vi "Init Digitizers.vi"(6 "NI Cards":i32=3, 8 "Bypass 2nd Digitizer Init":bool, 9 "Digitizer Config":T3=enum."5-CH pulser w/ ann array", 10 "Main Digitizer":T2=enum."NI Digitizer", 11 "Digitizer Settings in":T1={"Digitizer delay (us) "=0.0, "rf points per line"=0, "lines per plane"=0, "Samp Rate (Hz)"=0.0, "Additional dig delay (us)"=0.0, "Voltage Scale"=0.0, "Pre-Looks"=0, "Offset delay (us)"=0.0, "bits A/D"=0, "Avg Num"=0, "DigTimeOut"=0.0, "Rel Dig Delay"=0.0, "Dig Ch"=0, "LeCroyCluster"={"LeCroy Channels"=[], "LC read pt offset"=0.0, "Sweep Avg"=FALSE}, "Main Digitizer"=enum."Acqiris Digitizer", "Dig Config"=enum."Single channel", "Digitizer ID Cluster"={"Acqiris/Alazar/SP ID"=[], "NI Instr Handles"=[], "LeCroy VISA"="", "GaGe Handle"={"Handle"=0, "Sample size"=0, "Resolution"=0, "Offset"=0, "Channels"=0, "Boards"=0}, "ATS Ref"="", "Acqiris Address"=[], "ADQRef"=refnum, "adq_cu_ptr"=refnum}, "Trigger Settings"={"Trig Source"=0, "Trig Coupling"=0, "Trig Slope"=0, "Level (mV)"=0.0}, "Bulk Acq"=FALSE, "Bulk Start Indexes"=[], "Data Ref RF"=refnum, "NI ID/Channel"=[], "Total Dig CH"=1, "Xtra Ann Trig delay (us)"=10.0, "Fix Z Delay?"=FALSE, "One Way Transmission?"=FALSE, "Data Ref Log"=refnum} {"Trigger Settings"."Trig Slope" items=["Positive", "Negative"]; "Trigger Settings"."Level (mV)" format="%.2f"; "Trigger Settings"."Trig Coupling" items=["DC 1 MOhm", "AC 1 MOhm", "DC 50 Ohm", "AC 50 Ohm"]; "Trigger Settings"."Trig Source" items=["Chan 1", "External"]; "Rel Dig Delay" format="%.2f"; "DigTimeOut" format="%.2f"; "Avg Num" min=1; "Offset delay (us)" format="%.2f"; "Additional dig delay (us)" format="%.2f"; "Digitizer delay (us)" format="%.2f"}) -> (0 "Bypass 2nd Digitizer Init":bool, 1 "Initialization Failed!!":bool, 3 "Digitizer Settings":T1={"Digitizer delay (us) "=0.0, "rf points per line"=0, "lines per plane"=0, "Samp Rate (Hz)"=0.0, "Additional dig delay (us)"=0.0, "Voltage Scale"=0.0, "Pre-Looks"=0, "Offset delay (us)"=0.0, "bits A/D"=0, "Avg Num"=0, "DigTimeOut"=0.0, "Rel Dig Delay"=0.0, "Dig Ch"=0, "LeCroyCluster"={"LeCroy Channels"=[], "LC read pt offset"=0.0, "Sweep Avg"=FALSE}, "Main Digitizer"=enum."Acqiris Digitizer", "Dig Config"=enum."Single channel", "Digitizer ID Cluster"={"Acqiris/Alazar/SP ID"=[], "NI Instr Handles"=[], "LeCroy VISA"="", "GaGe Handle"={"Handle"=0, "Sample size"=0, "Resolution"=0, "Offset"=0, "Channels"=0, "Boards"=0}, "ATS Ref"="", "Acqiris Address"=[], "ADQRef"=refnum, "adq_cu_ptr"=refnum}, "Trigger Settings"={"Trig Source"=0, "Trig Coupling"=0, "Trig Slope"=0, "Level (mV)"=0.0}, "Bulk Acq"=FALSE, "Bulk Start Indexes"=[], "Data Ref RF"=refnum, "NI ID/Channel"=[], "Total Dig CH"=1, "Xtra Ann Trig delay (us)"=10.0, "Fix Z Delay?"=FALSE, "One Way Transmission?"=FALSE, "Data Ref Log"=refnum} {"Trigger Settings"."Trig Slope" items=["Positive", "Negative"]; "Trigger Settings"."Level (mV)" format="%.2f"; "Trigger Settings"."Trig Coupling" items=["DC 1 MOhm", "AC 1 MOhm", "DC 50 Ohm", "AC 50 Ohm"]; "Trigger Settings"."Trig Source" items=["Chan 1", "External"]; "Rel Dig Delay" format="%.2f"; "DigTimeOut" format="%.2f"; "Avg Num" min=1; "Offset delay (us)" format="%.2f"; "Additional dig delay (us)" format="%.2f"; "Digitizer delay (us)" format="%.2f"})   [LabVIEW 2022 SP3]
uses:
  -DigitizerRoutines/Digitizer.ctl
  -DigitizerRoutines/DigConfig.ctl
  -DigitizerRoutines/DigitizerSettings.ctl
  -DigitizerRoutines/DigitizerID.ctl
  C:/Windows/System32/ADQAPI_dotNet_helper.dll
  <instrlib>/niScope/Controls/niScope input clock source.ctl
  <instrlib>/Acqiris Dx/Acqiris Dx.lvlib
  <instrlib>/Acqiris Bx/Acqiris Bx.lvlib
  <instrlib>/LeCroy Wave Series/LeCroy Wave Series.lvlib
panel:
  out "error out":errorcluster
  in  "error in (no error)":errorcluster
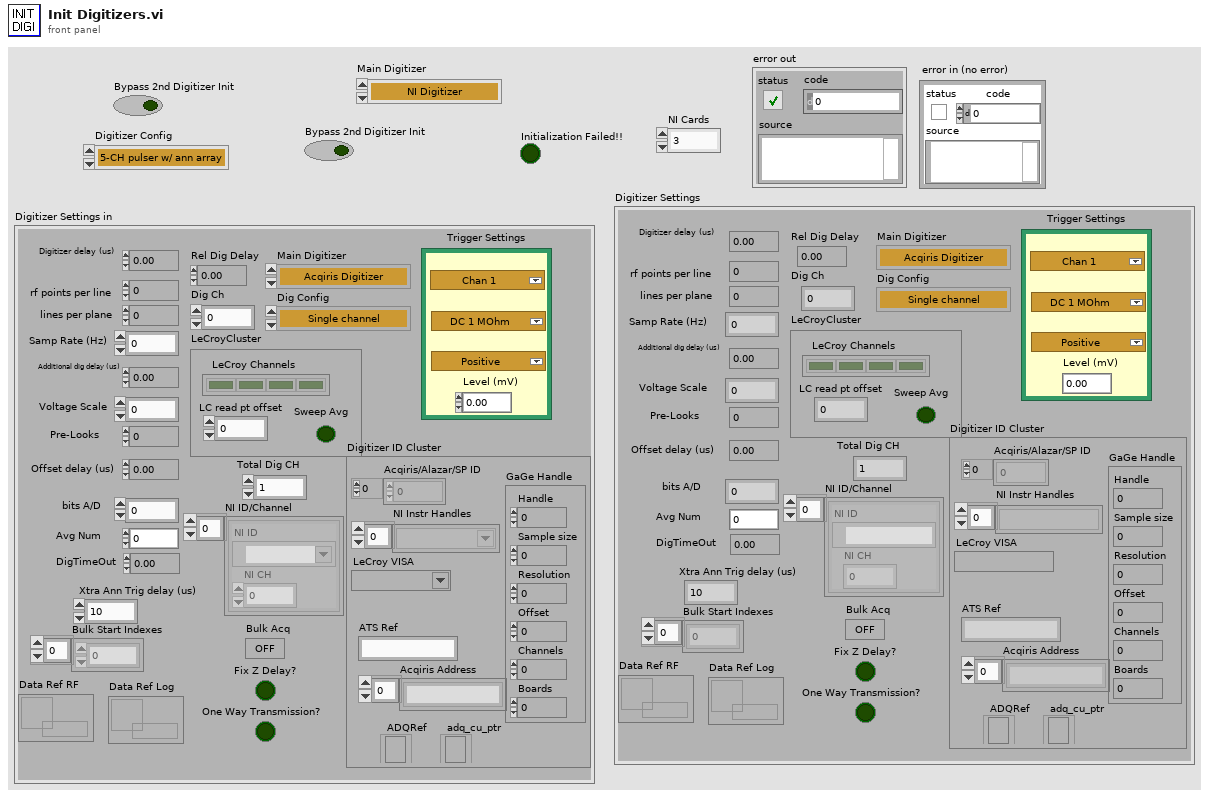
[diagram p1: front panel]
types:
  T1 = typedef "DigitizerSettings.ctl" = cluster{"Digitizer delay (us) ":dbl, "rf points per line":i32, "lines per plane":i32, "Samp Rate (Hz)":dbl, "Additional dig delay (us)":dbl, "Voltage Scale":dbl, "Pre-Looks":i32, "Offset delay (us)":dbl, "bits A/D":i8, "Avg Num":i32, "DigTimeOut":sgl, "Rel Dig Delay":sgl, "Dig Ch":i32, "LeCroyCluster":cluster{"LeCroy Channels":bool[], "LC read pt offset":dbl, "Sweep Avg":bool}, "Main Digitizer":T2, "Dig Config":T3, "Digitizer ID Cluster":T4, "Trigger Settings":cluster{"Trig Source":u16, "Trig Coupling":u16, "Trig Slope":u16, "Level (mV)":dbl}, "Bulk Acq":bool, "Bulk Start Indexes":i32[], "Data Ref RF":refnum<data-value>, "NI ID/Channel":cluster{"NI ID":refnum<k15>, "NI CH":i32}[], "Total Dig CH":i32, "Xtra Ann Trig delay (us)":dbl, "Fix Z Delay?":bool, "One Way Transmission?":bool, "Data Ref Log":refnum<data-value>}
  T2 = typedef "Digitizer.ctl" = enum16{"Acqiris Digitizer", "NI Digitizer", "LeCroy", "GaGe", "AlazarTech", "No Digitizer", "Teledyne"}
  T3 = typedef "DigConfig.ctl" = enum16{"Single channel", "2 Chans w/ 2 Acqiris", "2 Chans w/ 1 Acqiris", "5-CH Pulser New", "5-CH pulser w/ ann array", "5-pass style ann array", "Empty"}
  T4 = typedef "DigitizerID.ctl" = cluster{"Acqiris/Alazar/SP ID":u32[], "NI Instr Handles":refnum<k15>[], "LeCroy VISA":refnum<visa-resource-name>, "GaGe Handle":cluster{"Handle":u32, "Sample size":u32, "Resolution":i32, "Offset":i32, "Channels":u32, "Boards":u32}, "ATS Ref":string, "Acqiris Address":string[], "ADQRef":refnum<k24>, "adq_cu_ptr":refnum<k24>}
  T5 = typedef "niScope input clock source.ctl" = u16
  T6 = cluster{"instrument handle out":refnum<k15>, i32}
  T7 = cluster{"instrument handle out":refnum<k15>, i32}[]
  T8 = cluster{"Handle":u32, "Sample size":u32, "Resolution":i32, "Offset":i32, "Channels":u32, "Boards":u32}
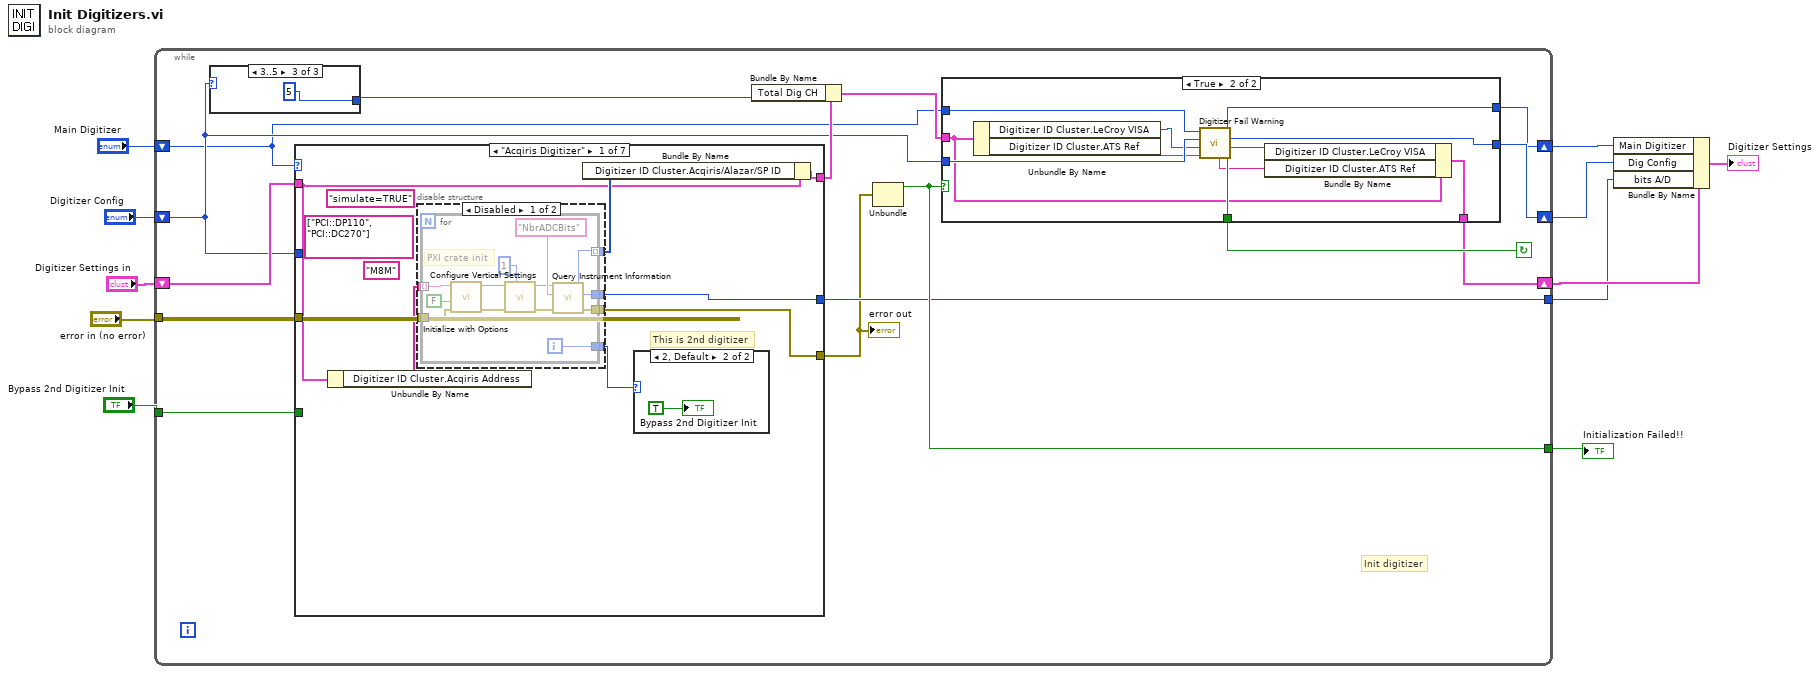
[diagram p0: block diagram]
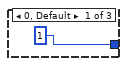
[diagram p2: hidden frame]
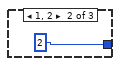
[diagram p3: hidden frame]
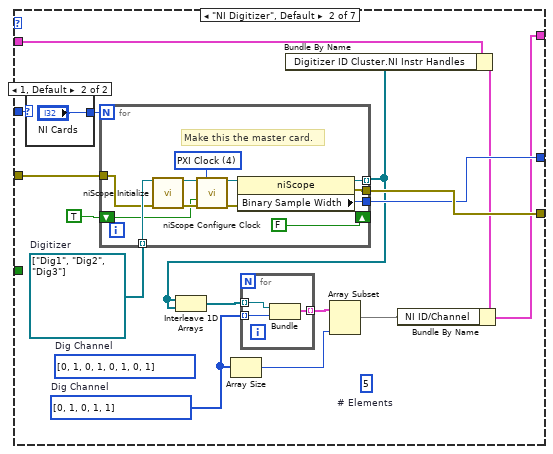
[diagram p7: hidden frame]
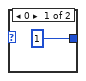
[diagram p8: hidden frame]
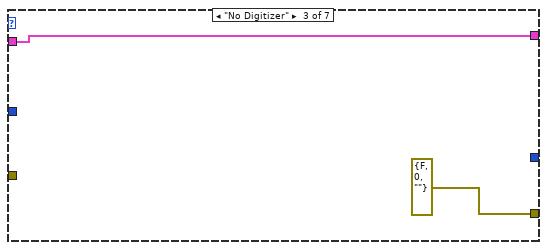
[diagram p9: hidden frame]
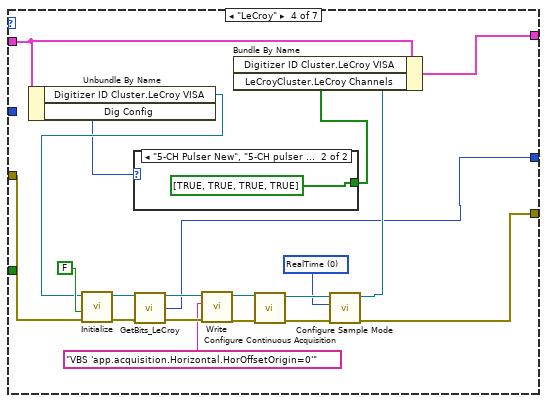
[diagram p10: hidden frame]
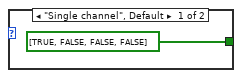
[diagram p11: hidden frame]
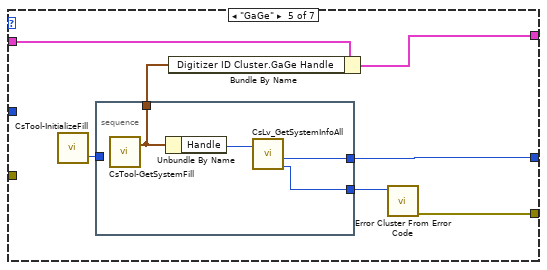
[diagram p12: hidden frame]
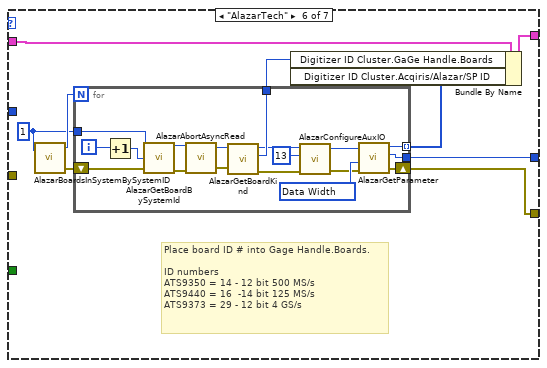
[diagram p13: hidden frame]
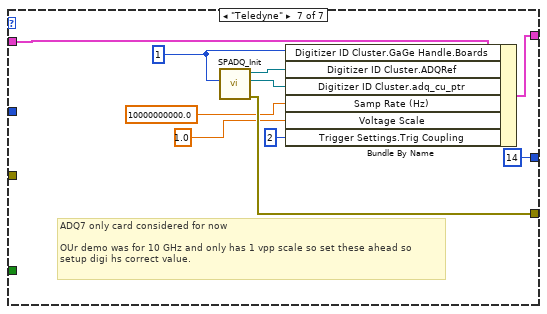
[diagram p14: hidden frame]
diagram:
  n1 = while {
    tunnel: "Bypass 2nd Digitizer Init" -> [w26]
    tunnel: "error in (no error)" -> [w24]
    tunnel: [w23] -> w8
    shift-right: [w17] -> w5
    shift-left: "Digitizer Settings in" -> [w25]
    shift-right: [w21] -> w2
    shift-left: "Digitizer Config" -> [w13]
    shift-right: [w20] -> w3
    shift-left: "Main Digitizer" -> [w12]
    tunnel: [w19] -> w1
    stop <- w22 continue-if-true
    # "Init digitizer"
    n2 = case shown="3..5" w13 {
      tunnel: [1 2 5] -> w14
      frame 0, Default {
      }
      frame 1, 2 {
      }
      frame 3..5 {
      }
    }
    n3 = case shown="\"Acqiris Digitizer\"" w12 {
      tunnel: [w50 w83 _ w110 w136 w146 u32 14 ("Sample Bits")] -> w19
      tunnel: w26 -> [_ _ _ _ _ _ _]
      tunnel: w13 -> [_ w88 _ _ _ _ _]
      tunnel: w25 -> [w49 w86 w106 w114 w134 w148 w175]
      tunnel: [w52 w78 w106 w115 w130 w149 w177] -> w16
      tunnel: [w47 w85 errorcluster {"status"=FALSE, "code"=0, "source"=""} ("error IO") w112 w131 w147 w171] -> w18
      tunnel: w24 -> [w46 w84 _ w113 _ _ _]
      frame "Acqiris Digitizer" {
        (unwired) "M8M" ("Options String (null string)")
        (unwired) string[] ["PCI::DP110", "PCI::DC270"]
        (unwired) "simulate=TRUE" ("Options String (null string)")
        # "This is 2nd digitizer"
        n4 = Unbundle By Name(w49) -> ("Digitizer ID Cluster.Acqiris Address"=w48:string[])
        n5 = disable-structure shown="Disabled" {
          disable-tunnel: [w58 _] -> w51
          disable-tunnel: [w57 _] -> w50
          disable-tunnel: w48 -> [w56 _]
          disable-tunnel: [w55 _] -> w47
          disable-tunnel: w46 -> [w54 _]
          disable-tunnel: [w53 _] -> w45
          frame Disabled {
            n6 = for {
              tunnel: [w64] -> w58 mode=indexing
              tunnel: w56 -> [w67] mode=indexing
              tunnel: [w62] -> w57
              tunnel: [w61] -> w55
              tunnel: w54 -> [w60]
              tunnel: [w59] -> w53
              i -> [w59]
              # "PXI crate init"
              n7 = call <instrlib>:"Initialize with Options.vi"("Resource Name (PCI::INSTR0)"=w67, "Reset (T: Reset)"=FALSE, "error in (no error)"=w60) -> ("Instrument ID"=w70:u32, "error out"=w69:errorcluster)  [unwired: 3 in, 2 out]
              n8 = call <instrlib>:"Configure Vertical Settings.vi"("Channel (1)"=1, "error in (no error)"=w69, "Instrument ID"=w70) -> ("error out"=w63:errorcluster, "dup Instrument ID"=w65:u32)  [unwired: 4 in, 3 out]
              n9 = call <instrlib>:"Query Instrument Information.vi"("Instrument ID"=w65, "Parameter String"="NbrADCBits", "error in (no error)"=w63) -> ("dup Instrument ID"=w64:u32, "Info Value (I32)"=w62:i32, "error out"=w61:errorcluster)  [unwired: 1 in, 3 out]
            }
          }
          frame Enabled {
          }
        }
        n10 = Bundle By Name(cluster=w49, "Digitizer ID Cluster.Acqiris/Alazar/SP ID"=w51) -> (w52:T1)
        n11 = case shown="2, Default" w45 {
          frame 0, 1 {
          }
          frame 2, Default {
            "Bypass 2nd Digitizer Init" <- TRUE ("Bypass 2nd Digitizer Init")
          }
        }
      }
      frame "NI Digitizer", Default {
        w73 = i32[] [0, 1, 0, 1, 1]  # Dig Channel
        (unwired) 5  # # Elements
        (unwired) i32[] [0, 1, 0, 1, 0, 1, 0, 1]  # Dig Channel
        w82 = refnum<k15>[] ["Dig1", "Dig2", "Dig3"]  # Digitizer
        n12 = case shown="1, Default" w88 {
          tunnel: [1 "NI Cards"] -> w87
          frame 0 {
          }
          frame 1, Default {
          }
        }
        n13 = for {
          N: w87 -> [_]
          tunnel: [w101] -> w74 mode=indexing
          tunnel: [w99] -> w83
          tunnel: w82 -> [w98] mode=indexing
          tunnel: [w97] -> w85
          tunnel: w84 -> [w96]
          shift-right: [FALSE] -> _
          shift-left: TRUE -> [w94]
          w103 = T5 4 items=["None"=0, "RTSI Clock"=1, "PFI 0"=6, "PFI 1"=2, "PFI 2"=3, "PXI Clock"=4, "External"=5, "Clock In"=7] ("input clock source")
          # "Make this the master card."
          n14 = call <instrlib>:"niScope Initialize.vi"("resource name"=w98, "error in"=w96) -> ("instrument handle"=w105:refnum<k15>, "error out"=w104:errorcluster)  [unwired: 2 in, 10 out]
          n15 = call <instrlib>:"niScope Configure Clock.vi"("instrument handle"=w105, "input clock source"=w103, "master enabled"=w94, "error in"=w104) -> ("instrument handle out"=w102:refnum<k15>, "error out"=w100:errorcluster)  [unwired: 2 in, 8 out]
          n16 = property class="niScope"(reference=w102, error in=w100) -> (reference out=w101:refnum<k15>, error out=w97:errorcluster, "Binary Sample Width"=w99:i32)
        }
        n17 = Interleave 1D Arrays(w74, w74) -> (w75:refnum<k15>[])
        n18 = Array Size(array=w73) -> (size(s)=w76:i32)
        n19 = for {
          tunnel: w75 -> [w91] mode=indexing
          tunnel: w73 -> [w90] mode=indexing
          tunnel: [w89] -> w81 mode=indexing
          n20 = Bundle("instrument handle out"=w91, w90) -> (w89:T6)  [unwired: 1 in]
        }
        n21 = Bundle By Name(cluster=w86, "Digitizer ID Cluster.NI Instr Handles"=w74) -> (w80:T1)
        n22 = Array Subset(array=w81, length=w76) -> (w79:T7)  [unwired: 1 in]
        n23 = Bundle By Name(cluster=w80, "NI ID/Channel"=w79) -> (w78:T1)
      }
      frame "No Digitizer" {
      }
      frame "LeCroy" {
        w122 = u16 0 items=["RealTime", "RIS", "Sequence", "Roll", "WaveStream"] ("Sample Mode (0: RealTime)")
        n24 = Unbundle By Name(w114) -> ("Digitizer ID Cluster.LeCroy VISA"=w111:refnum<visa-resource-name>, "Dig Config"=w109:T3)
        n25 = call <instrlib>:"Initialize.vi"("error in (no error)"=w113, "Reset? (T: Yes)"=FALSE, "VISA resource name"=w111) -> ("error out"=w125:errorcluster, "VISA resource name out"=w126:refnum<visa-resource-name>)  [unwired: 7 in]
        n26 = case shown="\"5-CH Pulser New\", \"5-CH pulser w/ ann array\"" w109 {
          tunnel: [bool[] [TRUE, FALSE, FALSE, FALSE] ("LeCroyCluster.LeCroy Channels") bool[] [TRUE, TRUE, TRUE, TRUE] ("LeCroyCluster.LeCroy Channels")] -> w108
          frame "Single channel", Default {
          }
          frame "5-CH Pulser New", "5-CH pulser w/ ann array" {
          }
        }
        n27 = call "GetBits_LeCroy.vi"("VISA resource name"=w126, "error in (no error)"=w125) -> ("VISA resource name out"=w118:refnum<visa-resource-name>, "Nom_Bits"=w110:i16, "error out"=w119:errorcluster)  [unwired: 11 in]
        n28 = call <instrlib>:"Write.vi"("error in (no error)"=w119, "Write Buffer"="VBS 'app.acquisition.Horizontal.HorOffsetOrigin=0'", "VISA resource name"=w118) -> ("error out"=w120:errorcluster, "VISA resource name out"=w121:refnum<visa-resource-name>)  [unwired: 6 in, 1 out]
        n29 = call <instrlib>:"Configure Continuous Acquisition.vi"("error in (no error)"=w120, "VISA resource name"=w121) -> ("error out"=w124:errorcluster, "VISA resource name out"=w123:refnum<visa-resource-name>)  [unwired: 8 in]
        n30 = call <instrlib>:"Configure Sample Mode.vi"("error in (no error)"=w124, "Sample Mode (0: RealTime)"=w122, "VISA resource name"=w123) -> ("error out"=w112:errorcluster, "VISA resource name out"=w116:refnum<visa-resource-name>)  [unwired: 7 in]
        n31 = Bundle By Name(cluster=w114, "Digitizer ID Cluster.LeCroy VISA"=w116, "LeCroyCluster.LeCroy Channels"=w108) -> (w115:T1)
      }
      frame "GaGe" {
        n32 = call "CsTool-InitializeFill.vi"() -> ("Error Code"=w135:i32)  [unwired: 1 out]
        n33 = stacked-sequence {
          tunnel: [w139] -> w136
          tunnel: w135 -> [_]
          tunnel: [w138] -> w133
          tunnel: [w137] -> w132
          frame #0 {
            n34 = call "CsTool-GetSystemFill.vi"() -> ("Handle Cluster"=w138:T8)  [unwired: 4 in, 1 out]
            n35 = Unbundle By Name(w138) -> ("Handle"=w140:u32)
            n36 = call "CsLv_GetSystemInfoAll.vi"("Handle"=w140) -> ("Sample Bits"=w139:u32, "Error Code"=w137:i32)  [unwired: 5 out]
          }
        }
        n37 = Bundle By Name(cluster=w134, "Digitizer ID Cluster.GaGe Handle"=w133) -> (w130:T1)
        n38 = call <vilib>:"Error Cluster From Error Code.vi"("error code (0)"=w132) -> ("error out"=w131:errorcluster)  [unwired: 8 in]
      }
      frame "AlazarTech" {
        w143 = u32 1 ("System ID")
        # "Place board ID # into Gage Handle.Boards.\n\nID numbers\nATS9350 = 14 - 12 bit 500 MS/s\nATS9440 = 16  -14 bit 125 MS/s\nATS9373 = 29 - 12 bit 4 GS/s"
        n39 = call "AlazarBoardsInSystemBySystemID.vi"("System ID"=w143) -> ("Board Count"=w144:u32, "error out"=w145:errorcluster)  [unwired: 1 in, 1 out]
        n40 = for {
          N: w144 -> [_]
          tunnel: [w167] -> w142 mode=indexing
          tunnel: [w164] -> w146
          shift-right: [w165] -> w147
          shift-left: w145 -> [w161]
          tunnel: w143 -> [w158]
          tunnel: [w155] -> w141
          i -> [w160]
          w166 = u32 268435465 items=["Data Width"=268435465, "Set/Get Async BuffSize"=268435513, "Set/Get Async Buffcount"=268435520, "Get Data Format"=268435522, "Get Samples Per Timestamp Clock"=268435524, "Get Records Captured"=268435525, "Get Async Buffers Pending"=268435536, "Get Async Buffers Pending Full"=268435537, "Get Async Buffers Pending Empty"=268435538, "ECC Mode"=268435528, "Get Aux Input Level"=268435529, "Get Channels Per Board"=268435568, "Pack Mode"=268435570, "Get FPGA Temperature"=268435584] ("Parameter")
          n41 = Increment(x=w160) -> (x+1=w159:i32)
          n42 = call "AlazarGetBoardBySystemId.vi"("error in (no error)"=w161, "Board ID"=w159, "System ID"=w158) -> ("error out"=w162:errorcluster, "Handle"=w163:u64)  [unwired: 1 out]
          n43 = call "AlazarAbortAsyncRead.vi"("Handle"=w163, "error in (no error)"=w162) -> ("Handle"=w157:u64, "error out"=w156:errorcluster)  [unwired: 1 out]
          n44 = call "AlazarGetBoardKind.vi"("Handle"=w157, "error in (no error)"=w156) -> ("Handle"=w152:u64, "Board Kind"=w155:u32, "error out"=w151:errorcluster)  [unwired: 1 out]
          n45 = call "AlazarConfigureAuxIO.vi"("error in (no error)"=w151, "Mode"=u32 13, "Handle"=w152) -> ("error out"=w153:errorcluster, "Handle"=w154:u64)  [unwired: 1 in, 1 out]
          n46 = call "AlazarGetParameter.vi"("error in (no error)"=w153, "Parameter"=w166, "Handle"=w154) -> ("error out"=w165:errorcluster, "Value"=w164:i32, "Handle"=w167:u64)  [unwired: 1 in, 1 out]
        }
        n47 = Bundle By Name(cluster=w148, "Digitizer ID Cluster.GaGe Handle.Boards"=w141, "Digitizer ID Cluster.Acqiris/Alazar/SP ID"=w142) -> (w149:T1)
      }
      frame "Teledyne" {
        w174 = u32 1 ("Digitizer ID Cluster.GaGe Handle.Boards")
        # "ADQ7 only card considered for now\n\nOUr demo was for 10 GHz and only has 1 vpp scale so set these ahead so \nsetup digi hs correct value."
        n48 = call "SPADQ_Init.vi"("adq_num"=w174) -> ("error out"=w171:errorcluster, "adq_cu_ptr"=w172:refnum<k24>, "ADQAPI Ref"=w173:refnum<k24>)  [unwired: 7 in, 1 out]
        n49 = Bundle By Name(cluster=w175, "Digitizer ID Cluster.GaGe Handle.Boards"=w174, "Digitizer ID Cluster.ADQRef"=w173, "Digitizer ID Cluster.adq_cu_ptr"=w172, "Samp Rate (Hz)"=10000000000.0, "Voltage Scale"=1.0, "Trigger Settings.Trig Coupling"=u16 2) -> (w177:T1)
      }
    }
    "error out" <- w18
    n50 = Bundle By Name(cluster=w16, "Total Dig CH"=w14) -> (w15:T1)
    n51 = Unbundle(w18) -> ("status"=w23:bool)  [unwired: 2 out]
    n52 = case shown="True" w23 {
      selector: w23 -> [w33 _]
      tunnel: w13 -> [w31 w44]
      tunnel: w12 -> [w30 w43]
      tunnel: [w33 w42] -> w22
      tunnel: [w31 w37] -> w21
      tunnel: [w30 w41] -> w20
      tunnel: w15 -> [w32 w39]
      tunnel: [w32 w40] -> w17
      frame False {
      }
      frame True {
        n53 = Unbundle By Name(w39) -> ("Digitizer ID Cluster.LeCroy VISA"=w34:refnum<visa-resource-name>, "Digitizer ID Cluster.ATS Ref"=w35:string)
        n54 = call "Digitizer Fail Warning.vi"("ATS Ref"=w35, "Scope Address"=w34, "Digitizer Config"=w44, "Main Digitizer"=w43) -> ("Retry"=w42:bool, "Scope Address"=w36:refnum<visa-resource-name>, "Digitizer Config"=w37:i32, "Main Digitizer"=w41:T2, "ATS Ref"=w38:string)  [unwired: 3 in]
        n55 = Bundle By Name(cluster=w39, "Digitizer ID Cluster.LeCroy VISA"=w36, "Digitizer ID Cluster.ATS Ref"=w38) -> (w40:T1)
      }
    }
  }
  "Initialization Failed!!" <- w8
  n56 = Bundle By Name(cluster=w5, "Main Digitizer"=w3, "Dig Config"=w2, "bits A/D"=w1) -> (→"Digitizer Settings":T1)
